vi "controller.vi"(11 "Shared_strings":string[][](array[string])) -> ()   [LabVIEW 2018]
uses:
  Global Variables.vi
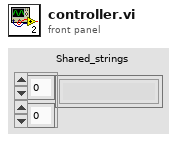
[diagram p1: front panel]
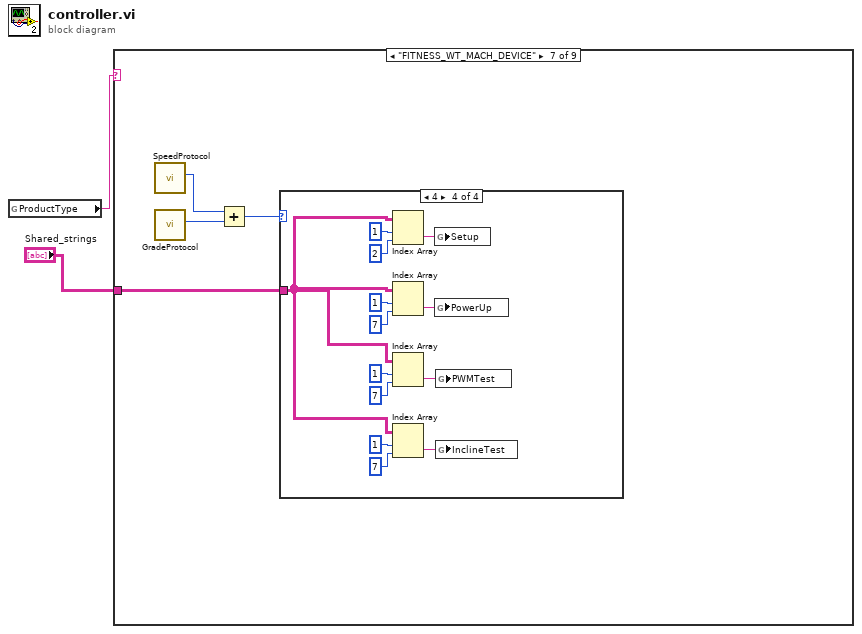
[diagram p0: block diagram]
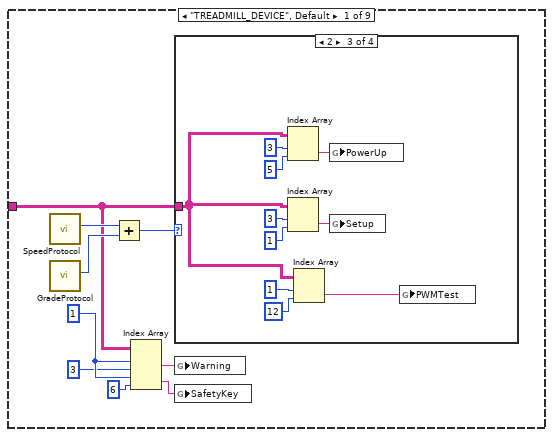
[diagram p2: hidden frame]
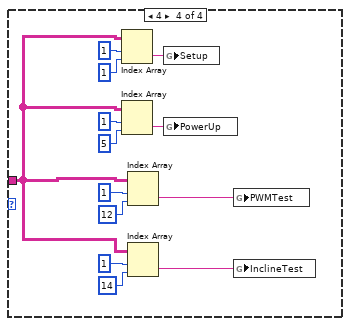
[diagram p5: hidden frame]
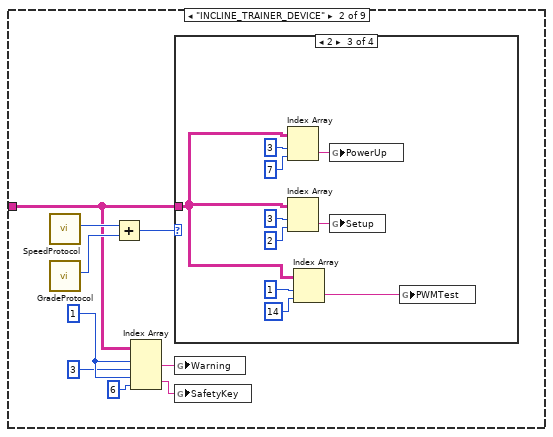
[diagram p6: hidden frame]
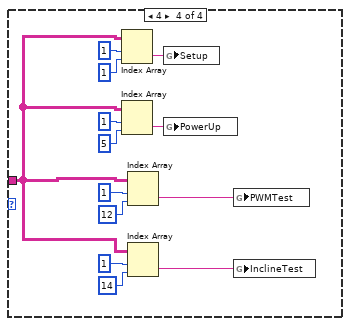
[diagram p9: hidden frame]
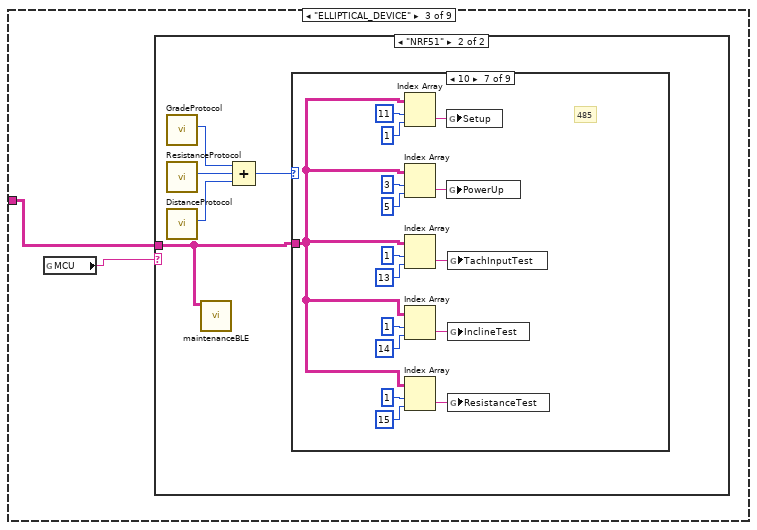
[diagram p10: hidden frame]
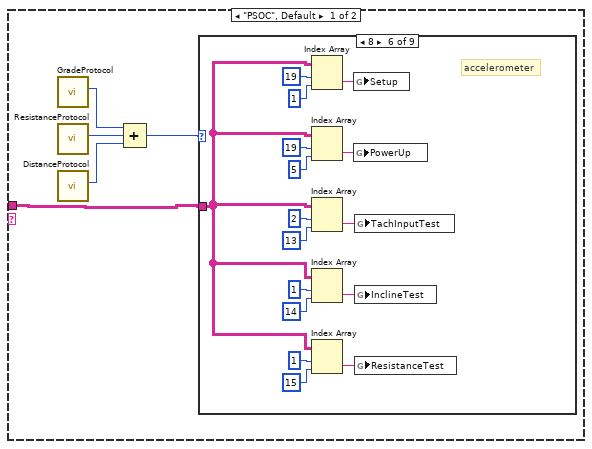
[diagram p11: hidden frame]
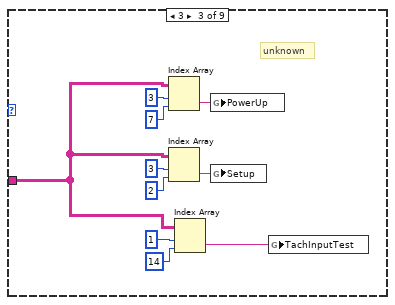
[diagram p14: hidden frame]
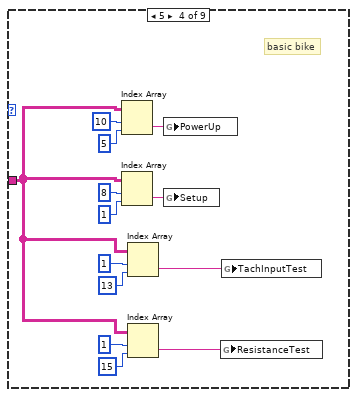
[diagram p15: hidden frame]
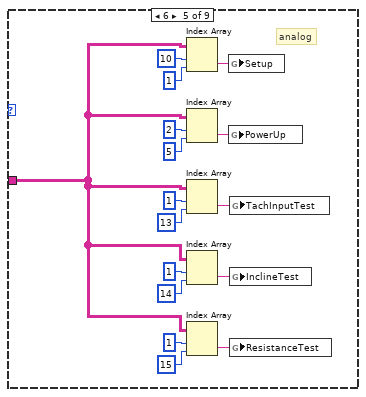
[diagram p16: hidden frame]
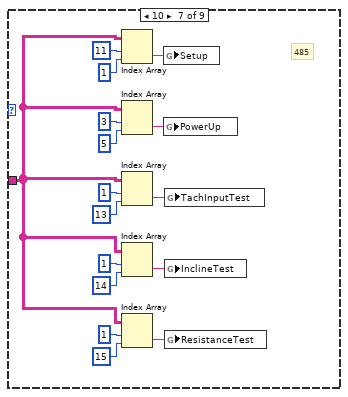
[diagram p17: hidden frame]
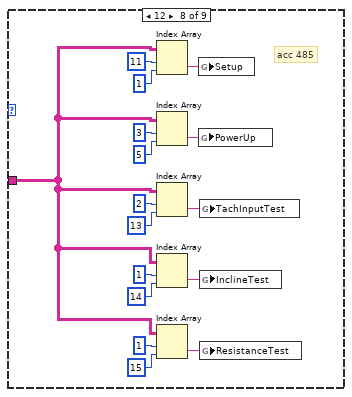
[diagram p18: hidden frame]
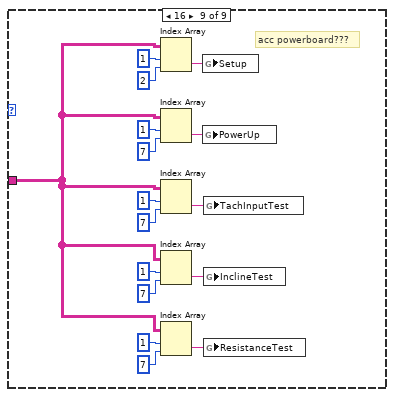
[diagram p19: hidden frame]
diagram:
  n1 = global read "Global Variables.vi" "ProductType"() -> (w1:string)
  n2 = case shown="\"FITNESS_WT_MACH_DEVICE\"" w1 {
    tunnel: "Shared_strings" -> [w3 w35 w68 w286 w406 w449 w667 w694 w913]
    frame "TREADMILL_DEVICE", Default {
      w8 = 1
      n3 = call "SpeedProtocol.vi"() -> ("output 1"=w11:i32)  [unwired: 9 in, 2 out]
      n4 = call "GradeProtocol.vi"() -> ("output 1"=w10:i32)  [unwired: 9 in, 2 out]
      n5 = Add(x=w11, y=w10) -> (x+y=w9:i32)
      n6 = Index Array(array=w3, index (row) #1=w8, index (col) #1=3, index (row) #2=w8, index (col) #2=6) -> (element #1=w5:string, element #2=w4:string)
      n7 = case shown="2" w9 {
        tunnel: w3 -> [_ _ w12 w22]
        frame 0, Default {
        }
        frame 1 {
        }
        frame 2 {
          n8 = Index Array(array=w12, index (row)=3, index (col)=5 ("disabled index (col)")) -> (element=w16:string)
          n9 = Index Array(array=w12, index (row)=3, index (col)=1 ("disabled index (col)")) -> (element=w21:string)
          n10 = Index Array(array=w12, index (row)=1, index (col)=12 ("disabled index (col)")) -> (element=w13:string)
          n11 = global write "Global Variables.vi" "PowerUp"(w16) -> ()
          n12 = global write "Global Variables.vi" "Setup"(w21) -> ()
          n13 = global write "Global Variables.vi" "PWMTest"(w13) -> ()
        }
        frame 4 {
          n14 = Index Array(array=w22, index (row)=1, index (col)=1 ("disabled index (col)")) -> (element=w34:string)
          n15 = Index Array(array=w22, index (row)=1, index (col)=5 ("disabled index (col)")) -> (element=w29:string)
          n16 = Index Array(array=w22, index (row)=1, index (col)=12 ("disabled index (col)")) -> (element=w26:string)
          n17 = Index Array(array=w22, index (row)=1, index (col)=14 ("disabled index (col)")) -> (element=w25:string)
          n18 = global write "Global Variables.vi" "Setup"(w34) -> ()
          n19 = global write "Global Variables.vi" "PowerUp"(w29) -> ()
          n20 = global write "Global Variables.vi" "PWMTest"(w26) -> ()
          n21 = global write "Global Variables.vi" "InclineTest"(w25) -> ()
        }
      }
      n22 = global write "Global Variables.vi" "Warning"(w5) -> ()
      n23 = global write "Global Variables.vi" "SafetyKey"(w4) -> ()
    }
    frame "INCLINE_TRAINER_DEVICE" {
      w40 = 1
      n24 = call "SpeedProtocol.vi"() -> ("output 1"=w43:i32)  [unwired: 9 in, 2 out]
      n25 = call "GradeProtocol.vi"() -> ("output 1"=w42:i32)  [unwired: 9 in, 2 out]
      n26 = Add(x=w43, y=w42) -> (x+y=w41:i32)
      n27 = Index Array(array=w35, index (row) #1=w40, index (col) #1=3, index (row) #2=w40, index (col) #2=6) -> (element #1=w36:string, element #2=w37:string)
      n28 = case shown="2" w41 {
        tunnel: w35 -> [_ _ w44 w54]
        frame 0, Default {
        }
        frame 1 {
        }
        frame 2 {
          n29 = Index Array(array=w44, index (row)=3, index (col)=7 ("disabled index (col)")) -> (element=w48:string)
          n30 = Index Array(array=w44, index (row)=3, index (col)=2 ("disabled index (col)")) -> (element=w53:string)
          n31 = Index Array(array=w44, index (row)=1, index (col)=14 ("disabled index (col)")) -> (element=w45:string)
          n32 = global write "Global Variables.vi" "PowerUp"(w48) -> ()
          n33 = global write "Global Variables.vi" "Setup"(w53) -> ()
          n34 = global write "Global Variables.vi" "PWMTest"(w45) -> ()
        }
        frame 4 {
          n35 = Index Array(array=w54, index (row)=1, index (col)=1 ("disabled index (col)")) -> (element=w66:string)
          n36 = Index Array(array=w54, index (row)=1, index (col)=5 ("disabled index (col)")) -> (element=w61:string)
          n37 = Index Array(array=w54, index (row)=1, index (col)=12 ("disabled index (col)")) -> (element=w58:string)
          n38 = Index Array(array=w54, index (row)=1, index (col)=14 ("disabled index (col)")) -> (element=w57:string)
          n39 = global write "Global Variables.vi" "Setup"(w66) -> ()
          n40 = global write "Global Variables.vi" "PowerUp"(w61) -> ()
          n41 = global write "Global Variables.vi" "PWMTest"(w58) -> ()
          n42 = global write "Global Variables.vi" "InclineTest"(w57) -> ()
        }
      }
      n43 = global write "Global Variables.vi" "Warning"(w36) -> ()
      n44 = global write "Global Variables.vi" "SafetyKey"(w37) -> ()
    }
    frame "ELLIPTICAL_DEVICE" {
      n45 = global read "Global Variables.vi" "MCU"() -> (w67:string)
      n46 = case shown="\"NRF51\"" w67 {
        tunnel: w68 -> [w70 w177]
        frame "PSOC", Default {
          n47 = call "GradeProtocol.vi"() -> ("output 1"=w71:i32)  [unwired: 9 in, 2 out]
          n48 = call "ResistanceProtocol.vi"() -> ("output 1"=w72:i32)  [unwired: 9 in, 2 out]
          n49 = call "DistanceProtocol.vi"() -> ("output 1"=w73:i32)  [unwired: 9 in, 2 out]
          n50 = Compound Arithmetic op=ADD(w71, w72, w73) -> (w69:i32)
          n51 = case shown="8" w69 {
            tunnel: w70 -> [_ _ w74 w84 w97 w113 w129 w145 w161]
            frame 0, Default {
            }
            frame 1 {
            }
            frame 3 {
              # "unknown"
              n52 = Index Array(array=w74, index (row)=3, index (col)=7 ("disabled index (col)")) -> (element=w78:string)
              n53 = Index Array(array=w74, index (row)=3, index (col)=2 ("disabled index (col)")) -> (element=w83:string)
              n54 = Index Array(array=w74, index (row)=1, index (col)=14 ("disabled index (col)")) -> (element=w75:string)
              n55 = global write "Global Variables.vi" "PowerUp"(w78) -> ()
              n56 = global write "Global Variables.vi" "Setup"(w83) -> ()
              n57 = global write "Global Variables.vi" "TachInputTest"(w75) -> ()
            }
            frame 5 {
              # "basic bike"
              n58 = Index Array(array=w84, index (row)=10, index (col)=5 ("disabled index (col)")) -> (element=w91:string)
              n59 = Index Array(array=w84, index (row)=8, index (col)=1 ("disabled index (col)")) -> (element=w96:string)
              n60 = Index Array(array=w84, index (row)=1, index (col)=13 ("disabled index (col)")) -> (element=w88:string)
              n61 = Index Array(array=w84, index (row)=1, index (col)=15 ("disabled index (col)")) -> (element=w87:string)
              n62 = global write "Global Variables.vi" "PowerUp"(w91) -> ()
              n63 = global write "Global Variables.vi" "Setup"(w96) -> ()
              n64 = global write "Global Variables.vi" "ResistanceTest"(w87) -> ()
              n65 = global write "Global Variables.vi" "TachInputTest"(w88) -> ()
            }
            frame 6 {
              # "analog"
              n66 = Index Array(array=w97, index (row)=10, index (col)=1 ("disabled index (col)")) -> (element=w112:string)
              n67 = Index Array(array=w97, index (row)=2, index (col)=5 ("disabled index (col)")) -> (element=w107:string)
              n68 = Index Array(array=w97, index (row)=1, index (col)=13 ("disabled index (col)")) -> (element=w104:string)
              n69 = Index Array(array=w97, index (row)=1, index (col)=14 ("disabled index (col)")) -> (element=w103:string)
              n70 = Index Array(array=w97, index (row)=1, index (col)=15 ("disabled index (col)")) -> (element=w98:string)
              n71 = global write "Global Variables.vi" "Setup"(w112) -> ()
              n72 = global write "Global Variables.vi" "PowerUp"(w107) -> ()
              n73 = global write "Global Variables.vi" "TachInputTest"(w104) -> ()
              n74 = global write "Global Variables.vi" "InclineTest"(w103) -> ()
              n75 = global write "Global Variables.vi" "ResistanceTest"(w98) -> ()
            }
            frame 8 {
              # "accelerometer"
              n76 = Index Array(array=w113, index (row)=19, index (col)=1 ("disabled index (col)")) -> (element=w128:string)
              n77 = Index Array(array=w113, index (row)=19, index (col)=5 ("disabled index (col)")) -> (element=w123:string)
              n78 = Index Array(array=w113, index (row)=2, index (col)=13 ("disabled index (col)")) -> (element=w120:string)
              n79 = Index Array(array=w113, index (row)=1, index (col)=14 ("disabled index (col)")) -> (element=w119:string)
              n80 = Index Array(array=w113, index (row)=1, index (col)=15 ("disabled index (col)")) -> (element=w114:string)
              n81 = global write "Global Variables.vi" "Setup"(w128) -> ()
              n82 = global write "Global Variables.vi" "PowerUp"(w123) -> ()
              n83 = global write "Global Variables.vi" "TachInputTest"(w120) -> ()
              n84 = global write "Global Variables.vi" "InclineTest"(w119) -> ()
              n85 = global write "Global Variables.vi" "ResistanceTest"(w114) -> ()
            }
            frame 10 {
              # "485"
              n86 = Index Array(array=w129, index (row)=11, index (col)=1 ("disabled index (col)")) -> (element=w144:string)
              n87 = Index Array(array=w129, index (row)=3, index (col)=5 ("disabled index (col)")) -> (element=w139:string)
              n88 = Index Array(array=w129, index (row)=1, index (col)=13 ("disabled index (col)")) -> (element=w136:string)
              n89 = Index Array(array=w129, index (row)=1, index (col)=14 ("disabled index (col)")) -> (element=w135:string)
              n90 = Index Array(array=w129, index (row)=1, index (col)=15 ("disabled index (col)")) -> (element=w130:string)
              n91 = global write "Global Variables.vi" "Setup"(w144) -> ()
              n92 = global write "Global Variables.vi" "PowerUp"(w139) -> ()
              n93 = global write "Global Variables.vi" "TachInputTest"(w136) -> ()
              n94 = global write "Global Variables.vi" "InclineTest"(w135) -> ()
              n95 = global write "Global Variables.vi" "ResistanceTest"(w130) -> ()
            }
            frame 12 {
              # "acc 485"
              n96 = Index Array(array=w145, index (row)=11, index (col)=1 ("disabled index (col)")) -> (element=w160:string)
              n97 = Index Array(array=w145, index (row)=3, index (col)=5 ("disabled index (col)")) -> (element=w155:string)
              n98 = Index Array(array=w145, index (row)=2, index (col)=13 ("disabled index (col)")) -> (element=w152:string)
              n99 = Index Array(array=w145, index (row)=1, index (col)=14 ("disabled index (col)")) -> (element=w151:string)
              n100 = Index Array(array=w145, index (row)=1, index (col)=15 ("disabled index (col)")) -> (element=w146:string)
              n101 = global write "Global Variables.vi" "Setup"(w160) -> ()
              n102 = global write "Global Variables.vi" "PowerUp"(w155) -> ()
              n103 = global write "Global Variables.vi" "TachInputTest"(w152) -> ()
              n104 = global write "Global Variables.vi" "InclineTest"(w151) -> ()
              n105 = global write "Global Variables.vi" "ResistanceTest"(w146) -> ()
            }
            frame 16 {
              # "acc powerboard???"
              n106 = Index Array(array=w161, index (row)=1, index (col)=2 ("disabled index (col)")) -> (element=w176:string)
              n107 = Index Array(array=w161, index (row)=1, index (col)=7 ("disabled index (col)")) -> (element=w171:string)
              n108 = Index Array(array=w161, index (row)=1, index (col)=7 ("disabled index (col)")) -> (element=w168:string)
              n109 = Index Array(array=w161, index (row)=1, index (col)=7 ("disabled index (col)")) -> (element=w167:string)
              n110 = Index Array(array=w161, index (row)=1, index (col)=7 ("disabled index (col)")) -> (element=w162:string)
              n111 = global write "Global Variables.vi" "Setup"(w176) -> ()
              n112 = global write "Global Variables.vi" "PowerUp"(w171) -> ()
              n113 = global write "Global Variables.vi" "TachInputTest"(w168) -> ()
              n114 = global write "Global Variables.vi" "InclineTest"(w167) -> ()
              n115 = global write "Global Variables.vi" "ResistanceTest"(w162) -> ()
            }
          }
        }
        frame "NRF51" {
          n116 = call "GradeProtocol.vi"() -> ("output 1"=w179:i32)  [unwired: 9 in, 2 out]
          n117 = call "ResistanceProtocol.vi"() -> ("output 1"=w180:i32)  [unwired: 9 in, 2 out]
          n118 = call "DistanceProtocol.vi"() -> ("output 1"=w181:i32)  [unwired: 9 in, 2 out]
          n119 = call "maintenanceBLE.vi"("Shared_strings"=w177) -> ()  [unwired: 11 in]
          n120 = Compound Arithmetic op=ADD(w179, w180, w181) -> (w178:i32)
          n121 = case shown="10" w178 {
            tunnel: w177 -> [_ _ w182 w192 w205 w221 w237 w253 w269]
            frame 0, Default {
            }
            frame 1 {
            }
            frame 3 {
              # "unknown"
              n122 = Index Array(array=w182, index (row)=3, index (col)=7 ("disabled index (col)")) -> (element=w186:string)
              n123 = Index Array(array=w182, index (row)=3, index (col)=2 ("disabled index (col)")) -> (element=w191:string)
              n124 = Index Array(array=w182, index (row)=1, index (col)=14 ("disabled index (col)")) -> (element=w183:string)
              n125 = global write "Global Variables.vi" "PowerUp"(w186) -> ()
              n126 = global write "Global Variables.vi" "Setup"(w191) -> ()
              n127 = global write "Global Variables.vi" "TachInputTest"(w183) -> ()
            }
            frame 5 {
              # "basic bike"
              n128 = Index Array(array=w192, index (row)=10, index (col)=5 ("disabled index (col)")) -> (element=w199:string)
              n129 = Index Array(array=w192, index (row)=8, index (col)=1 ("disabled index (col)")) -> (element=w204:string)
              n130 = Index Array(array=w192, index (row)=1, index (col)=13 ("disabled index (col)")) -> (element=w196:string)
              n131 = Index Array(array=w192, index (row)=1, index (col)=15 ("disabled index (col)")) -> (element=w195:string)
              n132 = global write "Global Variables.vi" "PowerUp"(w199) -> ()
              n133 = global write "Global Variables.vi" "Setup"(w204) -> ()
              n134 = global write "Global Variables.vi" "ResistanceTest"(w195) -> ()
              n135 = global write "Global Variables.vi" "TachInputTest"(w196) -> ()
            }
            frame 6 {
              # "analog"
              n136 = Index Array(array=w205, index (row)=10, index (col)=1 ("disabled index (col)")) -> (element=w220:string)
              n137 = Index Array(array=w205, index (row)=2, index (col)=5 ("disabled index (col)")) -> (element=w215:string)
              n138 = Index Array(array=w205, index (row)=1, index (col)=13 ("disabled index (col)")) -> (element=w212:string)
              n139 = Index Array(array=w205, index (row)=1, index (col)=14 ("disabled index (col)")) -> (element=w211:string)
              n140 = Index Array(array=w205, index (row)=1, index (col)=15 ("disabled index (col)")) -> (element=w206:string)
              n141 = global write "Global Variables.vi" "Setup"(w220) -> ()
              n142 = global write "Global Variables.vi" "PowerUp"(w215) -> ()
              n143 = global write "Global Variables.vi" "TachInputTest"(w212) -> ()
              n144 = global write "Global Variables.vi" "InclineTest"(w211) -> ()
              n145 = global write "Global Variables.vi" "ResistanceTest"(w206) -> ()
            }
            frame 8 {
              # "accelerometer"
              n146 = Index Array(array=w221, index (row)=19, index (col)=1 ("disabled index (col)")) -> (element=w236:string)
              n147 = Index Array(array=w221, index (row)=19, index (col)=5 ("disabled index (col)")) -> (element=w231:string)
              n148 = Index Array(array=w221, index (row)=2, index (col)=13 ("disabled index (col)")) -> (element=w228:string)
              n149 = Index Array(array=w221, index (row)=1, index (col)=14 ("disabled index (col)")) -> (element=w227:string)
              n150 = Index Array(array=w221, index (row)=1, index (col)=15 ("disabled index (col)")) -> (element=w222:string)
              n151 = global write "Global Variables.vi" "Setup"(w236) -> ()
              n152 = global write "Global Variables.vi" "PowerUp"(w231) -> ()
              n153 = global write "Global Variables.vi" "TachInputTest"(w228) -> ()
              n154 = global write "Global Variables.vi" "InclineTest"(w227) -> ()
              n155 = global write "Global Variables.vi" "ResistanceTest"(w222) -> ()
            }
            frame 10 {
              # "485"
              n156 = Index Array(array=w237, index (row)=11, index (col)=1 ("disabled index (col)")) -> (element=w252:string)
              n157 = Index Array(array=w237, index (row)=3, index (col)=5 ("disabled index (col)")) -> (element=w247:string)
              n158 = Index Array(array=w237, index (row)=1, index (col)=13 ("disabled index (col)")) -> (element=w244:string)
              n159 = Index Array(array=w237, index (row)=1, index (col)=14 ("disabled index (col)")) -> (element=w243:string)
              n160 = Index Array(array=w237, index (row)=1, index (col)=15 ("disabled index (col)")) -> (element=w238:string)
              n161 = global write "Global Variables.vi" "Setup"(w252) -> ()
              n162 = global write "Global Variables.vi" "PowerUp"(w247) -> ()
              n163 = global write "Global Variables.vi" "TachInputTest"(w244) -> ()
              n164 = global write "Global Variables.vi" "InclineTest"(w243) -> ()
              n165 = global write "Global Variables.vi" "ResistanceTest"(w238) -> ()
            }
            frame 12 {
              # "acc 485"
              n166 = Index Array(array=w253, index (row)=11, index (col)=1 ("disabled index (col)")) -> (element=w268:string)
              n167 = Index Array(array=w253, index (row)=3, index (col)=5 ("disabled index (col)")) -> (element=w263:string)
              n168 = Index Array(array=w253, index (row)=2, index (col)=13 ("disabled index (col)")) -> (element=w260:string)
              n169 = Index Array(array=w253, index (row)=1, index (col)=14 ("disabled index (col)")) -> (element=w259:string)
              n170 = Index Array(array=w253, index (row)=1, index (col)=15 ("disabled index (col)")) -> (element=w254:string)
              n171 = global write "Global Variables.vi" "Setup"(w268) -> ()
              n172 = global write "Global Variables.vi" "PowerUp"(w263) -> ()
              n173 = global write "Global Variables.vi" "TachInputTest"(w260) -> ()
              n174 = global write "Global Variables.vi" "InclineTest"(w259) -> ()
              n175 = global write "Global Variables.vi" "ResistanceTest"(w254) -> ()
            }
            frame 16 {
              # "acc powerboard???"
              n176 = Index Array(array=w269, index (row)=1, index (col)=2 ("disabled index (col)")) -> (element=w284:string)
              n177 = Index Array(array=w269, index (row)=1, index (col)=7 ("disabled index (col)")) -> (element=w279:string)
              n178 = Index Array(array=w269, index (row)=1, index (col)=7 ("disabled index (col)")) -> (element=w276:string)
              n179 = Index Array(array=w269, index (row)=1, index (col)=7 ("disabled index (col)")) -> (element=w275:string)
              n180 = Index Array(array=w269, index (row)=1, index (col)=7 ("disabled index (col)")) -> (element=w270:string)
              n181 = global write "Global Variables.vi" "Setup"(w284) -> ()
              n182 = global write "Global Variables.vi" "PowerUp"(w279) -> ()
              n183 = global write "Global Variables.vi" "TachInputTest"(w276) -> ()
              n184 = global write "Global Variables.vi" "InclineTest"(w275) -> ()
              n185 = global write "Global Variables.vi" "ResistanceTest"(w270) -> ()
            }
          }
        }
      }
    }
    frame "EXERCISE_BIKE_DEVICE" {
      n186 = global read "Global Variables.vi" "MCU"() -> (w285:string)
      n187 = case shown="\"PSOC\", Default" w285 {
        tunnel: w286 -> [w287 w346]
        frame "PSOC", Default {
          n188 = call "GradeProtocol.vi"() -> ("output 1"=w290:i32)  [unwired: 9 in, 2 out]
          n189 = call "ResistanceProtocol.vi"() -> ("output 1"=w289:i32)  [unwired: 9 in, 2 out]
          n190 = Compound Arithmetic op=ADD(w290, w289) -> (w288:i32)
          n191 = case shown="3" w288 {
            tunnel: w287 -> [_ _ w291 w301 w314 w330]
            frame 0, Default {
            }
            frame 1 {
            }
            frame 2 {
              # "incomplete"
              n192 = Index Array(array=w291, index (row)=3, index (col)=5 ("disabled index (col)")) -> (element=w295:string)
              n193 = Index Array(array=w291, index (row)=14, index (col)=1 ("disabled index (col)")) -> (element=w300:string)
              n194 = Index Array(array=w291, index (row)=1, index (col)=14 ("disabled index (col)")) -> (element=w292:string)
              n195 = global write "Global Variables.vi" "PowerUp"(w295) -> ()
              n196 = global write "Global Variables.vi" "Setup"(w300) -> ()
              n197 = global write "Global Variables.vi" "TachInputTest"(w292) -> ()
            }
            frame 3 {
              # "basic bike"
              n198 = Index Array(array=w301, index (row)=8, index (col)=1 ("disabled index (col)")) -> (element=w313:string)
              n199 = Index Array(array=w301, index (row)=8, index (col)=5 ("disabled index (col)")) -> (element=w308:string)
              n200 = Index Array(array=w301, index (row)=1, index (col)=13 ("disabled index (col)")) -> (element=w305:string)
              n201 = Index Array(array=w301, index (row)=1, index (col)=15 ("disabled index (col)")) -> (element=w304:string)
              n202 = global write "Global Variables.vi" "TachInputTest"(w305) -> ()
              n203 = global write "Global Variables.vi" "ResistanceTest"(w304) -> ()
              n204 = global write "Global Variables.vi" "Setup"(w313) -> ()
              n205 = global write "Global Variables.vi" "PowerUp"(w308) -> ()
            }
            frame 4 {
              # "analog"
              n206 = Index Array(array=w314, index (row)=9, index (col)=1 ("disabled index (col)")) -> (element=w329:string)
              n207 = Index Array(array=w314, index (row)=8, index (col)=5 ("disabled index (col)")) -> (element=w324:string)
              n208 = Index Array(array=w314, index (row)=1, index (col)=13 ("disabled index (col)")) -> (element=w321:string)
              n209 = Index Array(array=w314, index (row)=1, index (col)=14 ("disabled index (col)")) -> (element=w320:string)
              n210 = Index Array(array=w314, index (row)=1, index (col)=15 ("disabled index (col)")) -> (element=w315:string)
              n211 = global write "Global Variables.vi" "TachInputTest"(w321) -> ()
              n212 = global write "Global Variables.vi" "ResistanceTest"(w315) -> ()
              n213 = global write "Global Variables.vi" "Setup"(w329) -> ()
              n214 = global write "Global Variables.vi" "PowerUp"(w324) -> ()
              n215 = global write "Global Variables.vi" "InclineTest"(w320) -> ()
            }
            frame 8 {
              # "485"
              n216 = Index Array(array=w330, index (row)=11, index (col)=1 ("disabled index (col)")) -> (element=w345:string)
              n217 = Index Array(array=w330, index (row)=3, index (col)=5 ("disabled index (col)")) -> (element=w340:string)
              n218 = Index Array(array=w330, index (row)=1, index (col)=13 ("disabled index (col)")) -> (element=w337:string)
              n219 = Index Array(array=w330, index (row)=1, index (col)=14 ("disabled index (col)")) -> (element=w336:string)
              n220 = Index Array(array=w330, index (row)=1, index (col)=15 ("disabled index (col)")) -> (element=w331:string)
              n221 = global write "Global Variables.vi" "TachInputTest"(w337) -> ()
              n222 = global write "Global Variables.vi" "ResistanceTest"(w331) -> ()
              n223 = global write "Global Variables.vi" "Setup"(w345) -> ()
              n224 = global write "Global Variables.vi" "PowerUp"(w340) -> ()
              n225 = global write "Global Variables.vi" "InclineTest"(w336) -> ()
            }
          }
        }
        frame "NRF51" {
          n226 = call "GradeProtocol.vi"() -> ("output 1"=w349:i32)  [unwired: 9 in, 2 out]
          n227 = call "ResistanceProtocol.vi"() -> ("output 1"=w348:i32)  [unwired: 9 in, 2 out]
          n228 = call "maintenanceBLE.vi"("Shared_strings"=w346) -> ()  [unwired: 11 in]
          n229 = Compound Arithmetic op=ADD(w349, w348) -> (w347:i32)
          n230 = case shown="3" w347 {
            tunnel: w346 -> [_ _ w350 w360 w373 w389]
            frame 0, Default {
            }
            frame 1 {
            }
            frame 2 {
              # "incomplete"
              n231 = Index Array(array=w350, index (row)=3, index (col)=5 ("disabled index (col)")) -> (element=w354:string)
              n232 = Index Array(array=w350, index (row)=14, index (col)=1 ("disabled index (col)")) -> (element=w359:string)
              n233 = Index Array(array=w350, index (row)=1, index (col)=14 ("disabled index (col)")) -> (element=w351:string)
              n234 = global write "Global Variables.vi" "PowerUp"(w354) -> ()
              n235 = global write "Global Variables.vi" "Setup"(w359) -> ()
              n236 = global write "Global Variables.vi" "TachInputTest"(w351) -> ()
            }
            frame 3 {
              n237 = Index Array(array=w360, index (row)=8, index (col)=1 ("disabled index (col)")) -> (element=w372:string)
              n238 = Index Array(array=w360, index (row)=8, index (col)=5 ("disabled index (col)")) -> (element=w367:string)
              n239 = Index Array(array=w360, index (row)=1, index (col)=13 ("disabled index (col)")) -> (element=w364:string)
              n240 = Index Array(array=w360, index (row)=1, index (col)=15 ("disabled index (col)")) -> (element=w363:string)
              n241 = global write "Global Variables.vi" "TachInputTest"(w364) -> ()
              n242 = global write "Global Variables.vi" "ResistanceTest"(w363) -> ()
              n243 = global write "Global Variables.vi" "Setup"(w372) -> ()
              n244 = global write "Global Variables.vi" "PowerUp"(w367) -> ()
            }
            frame 4 {
              # "analog"
              n245 = Index Array(array=w373, index (row)=9, index (col)=1 ("disabled index (col)")) -> (element=w388:string)
              n246 = Index Array(array=w373, index (row)=8, index (col)=5 ("disabled index (col)")) -> (element=w383:string)
              n247 = Index Array(array=w373, index (row)=1, index (col)=13 ("disabled index (col)")) -> (element=w380:string)
              n248 = Index Array(array=w373, index (row)=1, index (col)=14 ("disabled index (col)")) -> (element=w379:string)
              n249 = Index Array(array=w373, index (row)=1, index (col)=15 ("disabled index (col)")) -> (element=w374:string)
              n250 = global write "Global Variables.vi" "TachInputTest"(w380) -> ()
              n251 = global write "Global Variables.vi" "ResistanceTest"(w374) -> ()
              n252 = global write "Global Variables.vi" "Setup"(w388) -> ()
              n253 = global write "Global Variables.vi" "PowerUp"(w383) -> ()
              n254 = global write "Global Variables.vi" "InclineTest"(w379) -> ()
            }
            frame 8 {
              # "485"
              n255 = Index Array(array=w389, index (row)=11, index (col)=1 ("disabled index (col)")) -> (element=w404:string)
              n256 = Index Array(array=w389, index (row)=3, index (col)=5 ("disabled index (col)")) -> (element=w399:string)
              n257 = Index Array(array=w389, index (row)=1, index (col)=13 ("disabled index (col)")) -> (element=w396:string)
              n258 = Index Array(array=w389, index (row)=1, index (col)=14 ("disabled index (col)")) -> (element=w395:string)
              n259 = Index Array(array=w389, index (row)=1, index (col)=15 ("disabled index (col)")) -> (element=w390:string)
              n260 = global write "Global Variables.vi" "TachInputTest"(w396) -> ()
              n261 = global write "Global Variables.vi" "ResistanceTest"(w390) -> ()
              n262 = global write "Global Variables.vi" "Setup"(w404) -> ()
              n263 = global write "Global Variables.vi" "PowerUp"(w399) -> ()
              n264 = global write "Global Variables.vi" "InclineTest"(w395) -> ()
            }
          }
        }
      }
    }
    frame "SPIN_BIKE_DEVICE" {
      n265 = global read "Global Variables.vi" "MCU"() -> (w405:string)
      n266 = case shown="\"NRF51\", Default" w405 {
        tunnel: w406 -> [w407 w429]
        frame "NRF51", Default {
          n267 = call "maintenanceBLE.vi"("Shared_strings"=w407) -> ()  [unwired: 11 in]
          n268 = call "SpeedProtocol.vi"() -> ("output 1"=w411:i32)  [unwired: 9 in, 2 out]
          n269 = call "GradeProtocol.vi"() -> ("output 1"=w410:i32)  [unwired: 9 in, 2 out]
          n270 = call "ResistanceProtocol.vi"() -> ("output 1"=w408:i32)  [unwired: 9 in, 2 out]
          n271 = Compound Arithmetic op=ADD(w411, w410, w408) -> (w409:i32)
          n272 = case shown="12" w409 {
            tunnel: w407 -> [_ w412]
            frame 0, Default {
            }
            frame 12 {
              # "RS485"
              n273 = Index Array(array=w412, index (row)=3, index (col)=5 ("disabled index (col)")) -> (element=w422:string)
              n274 = Index Array(array=w412, index (row)=1, index (col)=13 ("disabled index (col)")) -> (element=w419:string)
              n275 = Index Array(array=w412, index (row)=11, index (col)=1 ("disabled index (col)")) -> (element=w427:string)
              n276 = Index Array(array=w412, index (row)=1, index (col)=14 ("disabled index (col)")) -> (element=w418:string)
              n277 = Index Array(array=w412, index (row)=1, index (col)=15 ("disabled index (col)")) -> (element=w413:string)
              n278 = global write "Global Variables.vi" "PowerUp"(w422) -> ()
              n279 = global write "Global Variables.vi" "Setup"(w427) -> ()
              n280 = global write "Global Variables.vi" "TachInputTest"(w419) -> ()
              n281 = global write "Global Variables.vi" "InclineTest"(w418) -> ()
              n282 = global write "Global Variables.vi" "ResistanceTest"(w413) -> ()
            }
          }
        }
        frame "PSOC" {
          n283 = call "SpeedProtocol.vi"() -> ("output 1"=w432:i32)  [unwired: 9 in, 2 out]
          n284 = call "GradeProtocol.vi"() -> ("output 1"=w431:i32)  [unwired: 9 in, 2 out]
          n285 = call "ResistanceProtocol.vi"() -> ("output 1"=w428:i32)  [unwired: 9 in, 2 out]
          n286 = Compound Arithmetic op=ADD(w432, w431, w428) -> (w430:i32)
          n287 = case shown="12" w430 {
            tunnel: w429 -> [_ w433]
            frame 0, Default {
            }
            frame 12 {
              # "RS485"
              n288 = Index Array(array=w433, index (row)=16, index (col)=1 ("disabled index (col)")) -> (element=w448:string)
              n289 = Index Array(array=w433, index (row)=16, index (col)=5 ("disabled index (col)")) -> (element=w443:string)
              n290 = Index Array(array=w433, index (row)=1, index (col)=13 ("disabled index (col)")) -> (element=w440:string)
              n291 = Index Array(array=w433, index (row)=1, index (col)=14 ("disabled index (col)")) -> (element=w439:string)
              n292 = Index Array(array=w433, index (row)=1, index (col)=15 ("disabled index (col)")) -> (element=w434:string)
              n293 = global write "Global Variables.vi" "Setup"(w448) -> ()
              n294 = global write "Global Variables.vi" "PowerUp"(w443) -> ()
              n295 = global write "Global Variables.vi" "TachInputTest"(w440) -> ()
              n296 = global write "Global Variables.vi" "InclineTest"(w439) -> ()
              n297 = global write "Global Variables.vi" "ResistanceTest"(w434) -> ()
            }
          }
        }
      }
    }
    frame "VERTICAL_ELLIPTICAL_DEVICE" {
      n298 = global read "Global Variables.vi" "MCU"() -> (w450:string)
      n299 = case shown="\"NRF51\"" w450 {
        tunnel: w449 -> [w452 w559]
        frame "PSOC", Default {
          n300 = call "GradeProtocol.vi"() -> ("output 1"=w453:i32)  [unwired: 9 in, 2 out]
          n301 = call "ResistanceProtocol.vi"() -> ("output 1"=w454:i32)  [unwired: 9 in, 2 out]
          n302 = call "DistanceProtocol.vi"() -> ("output 1"=w455:i32)  [unwired: 9 in, 2 out]
          n303 = Compound Arithmetic op=ADD(w453, w454, w455) -> (w451:i32)
          n304 = case shown="8" w451 {
            tunnel: w452 -> [_ _ w456 w466 w479 w495 w511 w527 w543]
            frame 0, Default {
            }
            frame 1 {
            }
            frame 3 {
              # "unknown"
              n305 = Index Array(array=w456, index (row)=3, index (col)=7 ("disabled index (col)")) -> (element=w460:string)
              n306 = Index Array(array=w456, index (row)=3, index (col)=2 ("disabled index (col)")) -> (element=w465:string)
              n307 = Index Array(array=w456, index (row)=1, index (col)=14 ("disabled index (col)")) -> (element=w457:string)
              n308 = global write "Global Variables.vi" "PowerUp"(w460) -> ()
              n309 = global write "Global Variables.vi" "Setup"(w465) -> ()
              n310 = global write "Global Variables.vi" "TachInputTest"(w457) -> ()
            }
            frame 5 {
              # "basic bike"
              n311 = Index Array(array=w466, index (row)=10, index (col)=5 ("disabled index (col)")) -> (element=w473:string)
              n312 = Index Array(array=w466, index (row)=8, index (col)=1 ("disabled index (col)")) -> (element=w478:string)
              n313 = Index Array(array=w466, index (row)=1, index (col)=13 ("disabled index (col)")) -> (element=w470:string)
              n314 = Index Array(array=w466, index (row)=1, index (col)=15 ("disabled index (col)")) -> (element=w469:string)
              n315 = global write "Global Variables.vi" "PowerUp"(w473) -> ()
              n316 = global write "Global Variables.vi" "Setup"(w478) -> ()
              n317 = global write "Global Variables.vi" "ResistanceTest"(w469) -> ()
              n318 = global write "Global Variables.vi" "TachInputTest"(w470) -> ()
            }
            frame 6 {
              # "analog"
              n319 = Index Array(array=w479, index (row)=10, index (col)=1 ("disabled index (col)")) -> (element=w494:string)
              n320 = Index Array(array=w479, index (row)=2, index (col)=5 ("disabled index (col)")) -> (element=w489:string)
              n321 = Index Array(array=w479, index (row)=1, index (col)=13 ("disabled index (col)")) -> (element=w486:string)
              n322 = Index Array(array=w479, index (row)=1, index (col)=14 ("disabled index (col)")) -> (element=w485:string)
              n323 = Index Array(array=w479, index (row)=1, index (col)=15 ("disabled index (col)")) -> (element=w480:string)
              n324 = global write "Global Variables.vi" "Setup"(w494) -> ()
              n325 = global write "Global Variables.vi" "PowerUp"(w489) -> ()
              n326 = global write "Global Variables.vi" "TachInputTest"(w486) -> ()
              n327 = global write "Global Variables.vi" "InclineTest"(w485) -> ()
              n328 = global write "Global Variables.vi" "ResistanceTest"(w480) -> ()
            }
            frame 8 {
              # "accelerometer"
              n329 = Index Array(array=w495, index (row)=19, index (col)=1 ("disabled index (col)")) -> (element=w510:string)
              n330 = Index Array(array=w495, index (row)=19, index (col)=5 ("disabled index (col)")) -> (element=w505:string)
              n331 = Index Array(array=w495, index (row)=2, index (col)=13 ("disabled index (col)")) -> (element=w502:string)
              n332 = Index Array(array=w495, index (row)=1, index (col)=14 ("disabled index (col)")) -> (element=w501:string)
              n333 = Index Array(array=w495, index (row)=1, index (col)=15 ("disabled index (col)")) -> (element=w496:string)
              n334 = global write "Global Variables.vi" "Setup"(w510) -> ()
              n335 = global write "Global Variables.vi" "PowerUp"(w505) -> ()
              n336 = global write "Global Variables.vi" "TachInputTest"(w502) -> ()
              n337 = global write "Global Variables.vi" "InclineTest"(w501) -> ()
              n338 = global write "Global Variables.vi" "ResistanceTest"(w496) -> ()
            }
            frame 10 {
              # "485"
              n339 = Index Array(array=w511, index (row)=11, index (col)=1 ("disabled index (col)")) -> (element=w526:string)
              n340 = Index Array(array=w511, index (row)=3, index (col)=5 ("disabled index (col)")) -> (element=w521:string)
              n341 = Index Array(array=w511, index (row)=1, index (col)=13 ("disabled index (col)")) -> (element=w518:string)
              n342 = Index Array(array=w511, index (row)=1, index (col)=14 ("disabled index (col)")) -> (element=w517:string)
              n343 = Index Array(array=w511, index (row)=1, index (col)=15 ("disabled index (col)")) -> (element=w512:string)
              n344 = global write "Global Variables.vi" "Setup"(w526) -> ()
              n345 = global write "Global Variables.vi" "PowerUp"(w521) -> ()
              n346 = global write "Global Variables.vi" "TachInputTest"(w518) -> ()
              n347 = global write "Global Variables.vi" "InclineTest"(w517) -> ()
              n348 = global write "Global Variables.vi" "ResistanceTest"(w512) -> ()
            }
            frame 12 {
              # "acc 485"
              n349 = Index Array(array=w527, index (row)=11, index (col)=1 ("disabled index (col)")) -> (element=w542:string)
              n350 = Index Array(array=w527, index (row)=3, index (col)=5 ("disabled index (col)")) -> (element=w537:string)
              n351 = Index Array(array=w527, index (row)=2, index (col)=13 ("disabled index (col)")) -> (element=w534:string)
              n352 = Index Array(array=w527, index (row)=1, index (col)=14 ("disabled index (col)")) -> (element=w533:string)
              n353 = Index Array(array=w527, index (row)=1, index (col)=15 ("disabled index (col)")) -> (element=w528:string)
              n354 = global write "Global Variables.vi" "Setup"(w542) -> ()
              n355 = global write "Global Variables.vi" "PowerUp"(w537) -> ()
              n356 = global write "Global Variables.vi" "TachInputTest"(w534) -> ()
              n357 = global write "Global Variables.vi" "InclineTest"(w533) -> ()
              n358 = global write "Global Variables.vi" "ResistanceTest"(w528) -> ()
            }
            frame 16 {
              # "acc powerboard???"
              n359 = Index Array(array=w543, index (row)=1, index (col)=2 ("disabled index (col)")) -> (element=w558:string)
              n360 = Index Array(array=w543, index (row)=1, index (col)=7 ("disabled index (col)")) -> (element=w553:string)
              n361 = Index Array(array=w543, index (row)=1, index (col)=7 ("disabled index (col)")) -> (element=w550:string)
              n362 = Index Array(array=w543, index (row)=1, index (col)=7 ("disabled index (col)")) -> (element=w549:string)
              n363 = Index Array(array=w543, index (row)=1, index (col)=7 ("disabled index (col)")) -> (element=w544:string)
              n364 = global write "Global Variables.vi" "Setup"(w558) -> ()
              n365 = global write "Global Variables.vi" "PowerUp"(w553) -> ()
              n366 = global write "Global Variables.vi" "TachInputTest"(w550) -> ()
              n367 = global write "Global Variables.vi" "InclineTest"(w549) -> ()
              n368 = global write "Global Variables.vi" "ResistanceTest"(w544) -> ()
            }
          }
        }
        frame "NRF51" {
          n369 = call "GradeProtocol.vi"() -> ("output 1"=w561:i32)  [unwired: 9 in, 2 out]
          n370 = call "ResistanceProtocol.vi"() -> ("output 1"=w562:i32)  [unwired: 9 in, 2 out]
          n371 = call "DistanceProtocol.vi"() -> ("output 1"=w563:i32)  [unwired: 9 in, 2 out]
          n372 = call "maintenanceBLE.vi"("Shared_strings"=w559) -> ()  [unwired: 11 in]
          n373 = Compound Arithmetic op=ADD(w561, w562, w563) -> (w560:i32)
          n374 = case shown="10" w560 {
            tunnel: w559 -> [_ _ w564 w574 w587 w603 w619 w635 w651]
            frame 0, Default {
            }
            frame 1 {
            }
            frame 3 {
              # "unknown"
              n375 = Index Array(array=w564, index (row)=3, index (col)=7 ("disabled index (col)")) -> (element=w568:string)
              n376 = Index Array(array=w564, index (row)=3, index (col)=2 ("disabled index (col)")) -> (element=w573:string)
              n377 = Index Array(array=w564, index (row)=1, index (col)=14 ("disabled index (col)")) -> (element=w565:string)
              n378 = global write "Global Variables.vi" "PowerUp"(w568) -> ()
              n379 = global write "Global Variables.vi" "Setup"(w573) -> ()
              n380 = global write "Global Variables.vi" "TachInputTest"(w565) -> ()
            }
            frame 5 {
              # "basic bike"
              n381 = Index Array(array=w574, index (row)=10, index (col)=5 ("disabled index (col)")) -> (element=w581:string)
              n382 = Index Array(array=w574, index (row)=8, index (col)=1 ("disabled index (col)")) -> (element=w586:string)
              n383 = Index Array(array=w574, index (row)=1, index (col)=13 ("disabled index (col)")) -> (element=w578:string)
              n384 = Index Array(array=w574, index (row)=1, index (col)=15 ("disabled index (col)")) -> (element=w577:string)
              n385 = global write "Global Variables.vi" "PowerUp"(w581) -> ()
              n386 = global write "Global Variables.vi" "Setup"(w586) -> ()
              n387 = global write "Global Variables.vi" "ResistanceTest"(w577) -> ()
              n388 = global write "Global Variables.vi" "TachInputTest"(w578) -> ()
            }
            frame 6 {
              # "analog"
              n389 = Index Array(array=w587, index (row)=10, index (col)=1 ("disabled index (col)")) -> (element=w602:string)
              n390 = Index Array(array=w587, index (row)=2, index (col)=5 ("disabled index (col)")) -> (element=w597:string)
              n391 = Index Array(array=w587, index (row)=1, index (col)=13 ("disabled index (col)")) -> (element=w594:string)
              n392 = Index Array(array=w587, index (row)=1, index (col)=14 ("disabled index (col)")) -> (element=w593:string)
              n393 = Index Array(array=w587, index (row)=1, index (col)=15 ("disabled index (col)")) -> (element=w588:string)
              n394 = global write "Global Variables.vi" "Setup"(w602) -> ()
              n395 = global write "Global Variables.vi" "PowerUp"(w597) -> ()
              n396 = global write "Global Variables.vi" "TachInputTest"(w594) -> ()
              n397 = global write "Global Variables.vi" "InclineTest"(w593) -> ()
              n398 = global write "Global Variables.vi" "ResistanceTest"(w588) -> ()
            }
            frame 8 {
              # "accelerometer"
              n399 = Index Array(array=w603, index (row)=19, index (col)=1 ("disabled index (col)")) -> (element=w618:string)
              n400 = Index Array(array=w603, index (row)=19, index (col)=5 ("disabled index (col)")) -> (element=w613:string)
              n401 = Index Array(array=w603, index (row)=2, index (col)=13 ("disabled index (col)")) -> (element=w610:string)
              n402 = Index Array(array=w603, index (row)=1, index (col)=14 ("disabled index (col)")) -> (element=w609:string)
              n403 = Index Array(array=w603, index (row)=1, index (col)=15 ("disabled index (col)")) -> (element=w604:string)
              n404 = global write "Global Variables.vi" "Setup"(w618) -> ()
              n405 = global write "Global Variables.vi" "PowerUp"(w613) -> ()
              n406 = global write "Global Variables.vi" "TachInputTest"(w610) -> ()
              n407 = global write "Global Variables.vi" "InclineTest"(w609) -> ()
              n408 = global write "Global Variables.vi" "ResistanceTest"(w604) -> ()
            }
            frame 10 {
              # "485"
              n409 = Index Array(array=w619, index (row)=11, index (col)=1 ("disabled index (col)")) -> (element=w634:string)
              n410 = Index Array(array=w619, index (row)=3, index (col)=5 ("disabled index (col)")) -> (element=w629:string)
              n411 = Index Array(array=w619, index (row)=1, index (col)=13 ("disabled index (col)")) -> (element=w626:string)
              n412 = Index Array(array=w619, index (row)=1, index (col)=14 ("disabled index (col)")) -> (element=w625:string)
              n413 = Index Array(array=w619, index (row)=1, index (col)=15 ("disabled index (col)")) -> (element=w620:string)
              n414 = global write "Global Variables.vi" "Setup"(w634) -> ()
              n415 = global write "Global Variables.vi" "PowerUp"(w629) -> ()
              n416 = global write "Global Variables.vi" "TachInputTest"(w626) -> ()
              n417 = global write "Global Variables.vi" "InclineTest"(w625) -> ()
              n418 = global write "Global Variables.vi" "ResistanceTest"(w620) -> ()
            }
            frame 12 {
              # "acc 485"
              n419 = Index Array(array=w635, index (row)=11, index (col)=1 ("disabled index (col)")) -> (element=w650:string)
              n420 = Index Array(array=w635, index (row)=3, index (col)=5 ("disabled index (col)")) -> (element=w645:string)
              n421 = Index Array(array=w635, index (row)=2, index (col)=13 ("disabled index (col)")) -> (element=w642:string)
              n422 = Index Array(array=w635, index (row)=1, index (col)=14 ("disabled index (col)")) -> (element=w641:string)
              n423 = Index Array(array=w635, index (row)=1, index (col)=15 ("disabled index (col)")) -> (element=w636:string)
              n424 = global write "Global Variables.vi" "Setup"(w650) -> ()
              n425 = global write "Global Variables.vi" "PowerUp"(w645) -> ()
              n426 = global write "Global Variables.vi" "TachInputTest"(w642) -> ()
              n427 = global write "Global Variables.vi" "InclineTest"(w641) -> ()
              n428 = global write "Global Variables.vi" "ResistanceTest"(w636) -> ()
            }
            frame 16 {
              # "acc powerboard???"
              n429 = Index Array(array=w651, index (row)=1, index (col)=2 ("disabled index (col)")) -> (element=w666:string)
              n430 = Index Array(array=w651, index (row)=1, index (col)=7 ("disabled index (col)")) -> (element=w661:string)
              n431 = Index Array(array=w651, index (row)=1, index (col)=7 ("disabled index (col)")) -> (element=w658:string)
              n432 = Index Array(array=w651, index (row)=1, index (col)=7 ("disabled index (col)")) -> (element=w657:string)
              n433 = Index Array(array=w651, index (row)=1, index (col)=7 ("disabled index (col)")) -> (element=w652:string)
              n434 = global write "Global Variables.vi" "Setup"(w666) -> ()
              n435 = global write "Global Variables.vi" "PowerUp"(w661) -> ()
              n436 = global write "Global Variables.vi" "TachInputTest"(w658) -> ()
              n437 = global write "Global Variables.vi" "InclineTest"(w657) -> ()
              n438 = global write "Global Variables.vi" "ResistanceTest"(w652) -> ()
            }
          }
        }
      }
    }
    frame "FITNESS_WT_MACH_DEVICE" {
      n439 = call "SpeedProtocol.vi"() -> ("output 1"=w670:i32)  [unwired: 9 in, 2 out]
      n440 = call "GradeProtocol.vi"() -> ("output 1"=w669:i32)  [unwired: 9 in, 2 out]
      n441 = Add(x=w670, y=w669) -> (x+y=w668:i32)
      n442 = case shown="4" w668 {
        tunnel: w667 -> [_ _ w671 w681]
        frame 0, Default {
        }
        frame 1 {
        }
        frame 2 {
          n443 = Index Array(array=w671, index (row)=3, index (col)=7 ("disabled index (col)")) -> (element=w675:string)
          n444 = Index Array(array=w671, index (row)=3, index (col)=2 ("disabled index (col)")) -> (element=w680:string)
          n445 = Index Array(array=w671, index (row)=1, index (col)=14 ("disabled index (col)")) -> (element=w672:string)
          n446 = global write "Global Variables.vi" "PowerUp"(w675) -> ()
          n447 = global write "Global Variables.vi" "Setup"(w680) -> ()
          n448 = global write "Global Variables.vi" "PWMTest"(w672) -> ()
        }
        frame 4 {
          n449 = Index Array(array=w681, index (row)=1, index (col)=2 ("disabled index (col)")) -> (element=w693:string)
          n450 = Index Array(array=w681, index (row)=1, index (col)=7 ("disabled index (col)")) -> (element=w688:string)
          n451 = Index Array(array=w681, index (row)=1, index (col)=7 ("disabled index (col)")) -> (element=w685:string)
          n452 = Index Array(array=w681, index (row)=1, index (col)=7 ("disabled index (col)")) -> (element=w684:string)
          n453 = global write "Global Variables.vi" "Setup"(w693) -> ()
          n454 = global write "Global Variables.vi" "PowerUp"(w688) -> ()
          n455 = global write "Global Variables.vi" "PWMTest"(w685) -> ()
          n456 = global write "Global Variables.vi" "InclineTest"(w684) -> ()
        }
      }
    }
    frame "FREE_STRIDER_DEVICE" {
      n457 = global read "Global Variables.vi" "MCU"() -> (w695:string)
      n458 = case shown="\"NRF51\"" w695 {
        tunnel: w694 -> [w697 w804]
        frame "PSOC", Default {
          n459 = call "GradeProtocol.vi"() -> ("output 1"=w698:i32)  [unwired: 9 in, 2 out]
          n460 = call "ResistanceProtocol.vi"() -> ("output 1"=w699:i32)  [unwired: 9 in, 2 out]
          n461 = call "DistanceProtocol.vi"() -> ("output 1"=w700:i32)  [unwired: 9 in, 2 out]
          n462 = Compound Arithmetic op=ADD(w698, w699, w700) -> (w696:i32)
          n463 = case shown="8" w696 {
            tunnel: w697 -> [_ _ w701 w711 w724 w740 w756 w772 w788]
            frame 0, Default {
            }
            frame 1 {
            }
            frame 3 {
              # "unknown"
              n464 = Index Array(array=w701, index (row)=3, index (col)=7 ("disabled index (col)")) -> (element=w705:string)
              n465 = Index Array(array=w701, index (row)=3, index (col)=2 ("disabled index (col)")) -> (element=w710:string)
              n466 = Index Array(array=w701, index (row)=1, index (col)=14 ("disabled index (col)")) -> (element=w702:string)
              n467 = global write "Global Variables.vi" "PowerUp"(w705) -> ()
              n468 = global write "Global Variables.vi" "Setup"(w710) -> ()
              n469 = global write "Global Variables.vi" "TachInputTest"(w702) -> ()
            }
            frame 5 {
              # "basic bike"
              n470 = Index Array(array=w711, index (row)=10, index (col)=5 ("disabled index (col)")) -> (element=w718:string)
              n471 = Index Array(array=w711, index (row)=8, index (col)=1 ("disabled index (col)")) -> (element=w723:string)
              n472 = Index Array(array=w711, index (row)=1, index (col)=13 ("disabled index (col)")) -> (element=w715:string)
              n473 = Index Array(array=w711, index (row)=1, index (col)=15 ("disabled index (col)")) -> (element=w714:string)
              n474 = global write "Global Variables.vi" "PowerUp"(w718) -> ()
              n475 = global write "Global Variables.vi" "Setup"(w723) -> ()
              n476 = global write "Global Variables.vi" "ResistanceTest"(w714) -> ()
              n477 = global write "Global Variables.vi" "TachInputTest"(w715) -> ()
            }
            frame 6 {
              # "analog"
              n478 = Index Array(array=w724, index (row)=10, index (col)=1 ("disabled index (col)")) -> (element=w739:string)
              n479 = Index Array(array=w724, index (row)=2, index (col)=5 ("disabled index (col)")) -> (element=w734:string)
              n480 = Index Array(array=w724, index (row)=1, index (col)=13 ("disabled index (col)")) -> (element=w731:string)
              n481 = Index Array(array=w724, index (row)=1, index (col)=14 ("disabled index (col)")) -> (element=w730:string)
              n482 = Index Array(array=w724, index (row)=1, index (col)=15 ("disabled index (col)")) -> (element=w725:string)
              n483 = global write "Global Variables.vi" "Setup"(w739) -> ()
              n484 = global write "Global Variables.vi" "PowerUp"(w734) -> ()
              n485 = global write "Global Variables.vi" "TachInputTest"(w731) -> ()
              n486 = global write "Global Variables.vi" "InclineTest"(w730) -> ()
              n487 = global write "Global Variables.vi" "ResistanceTest"(w725) -> ()
            }
            frame 8 {
              # "accelerometer"
              n488 = Index Array(array=w740, index (row)=19, index (col)=1 ("disabled index (col)")) -> (element=w755:string)
              n489 = Index Array(array=w740, index (row)=19, index (col)=5 ("disabled index (col)")) -> (element=w750:string)
              n490 = Index Array(array=w740, index (row)=2, index (col)=13 ("disabled index (col)")) -> (element=w747:string)
              n491 = Index Array(array=w740, index (row)=1, index (col)=14 ("disabled index (col)")) -> (element=w746:string)
              n492 = Index Array(array=w740, index (row)=1, index (col)=15 ("disabled index (col)")) -> (element=w741:string)
              n493 = global write "Global Variables.vi" "Setup"(w755) -> ()
              n494 = global write "Global Variables.vi" "PowerUp"(w750) -> ()
              n495 = global write "Global Variables.vi" "TachInputTest"(w747) -> ()
              n496 = global write "Global Variables.vi" "InclineTest"(w746) -> ()
              n497 = global write "Global Variables.vi" "ResistanceTest"(w741) -> ()
            }
            frame 10 {
              # "485"
              n498 = Index Array(array=w756, index (row)=11, index (col)=1 ("disabled index (col)")) -> (element=w771:string)
              n499 = Index Array(array=w756, index (row)=3, index (col)=5 ("disabled index (col)")) -> (element=w766:string)
              n500 = Index Array(array=w756, index (row)=1, index (col)=13 ("disabled index (col)")) -> (element=w763:string)
              n501 = Index Array(array=w756, index (row)=1, index (col)=14 ("disabled index (col)")) -> (element=w762:string)
              n502 = Index Array(array=w756, index (row)=1, index (col)=15 ("disabled index (col)")) -> (element=w757:string)
              n503 = global write "Global Variables.vi" "Setup"(w771) -> ()
              n504 = global write "Global Variables.vi" "PowerUp"(w766) -> ()
              n505 = global write "Global Variables.vi" "TachInputTest"(w763) -> ()
              n506 = global write "Global Variables.vi" "InclineTest"(w762) -> ()
              n507 = global write "Global Variables.vi" "ResistanceTest"(w757) -> ()
            }
            frame 12 {
              # "acc 485"
              n508 = Index Array(array=w772, index (row)=11, index (col)=1 ("disabled index (col)")) -> (element=w787:string)
              n509 = Index Array(array=w772, index (row)=3, index (col)=5 ("disabled index (col)")) -> (element=w782:string)
              n510 = Index Array(array=w772, index (row)=2, index (col)=13 ("disabled index (col)")) -> (element=w779:string)
              n511 = Index Array(array=w772, index (row)=1, index (col)=14 ("disabled index (col)")) -> (element=w778:string)
              n512 = Index Array(array=w772, index (row)=1, index (col)=15 ("disabled index (col)")) -> (element=w773:string)
              n513 = global write "Global Variables.vi" "Setup"(w787) -> ()
              n514 = global write "Global Variables.vi" "PowerUp"(w782) -> ()
              n515 = global write "Global Variables.vi" "TachInputTest"(w779) -> ()
              n516 = global write "Global Variables.vi" "InclineTest"(w778) -> ()
              n517 = global write "Global Variables.vi" "ResistanceTest"(w773) -> ()
            }
            frame 16 {
              # "acc powerboard???"
              n518 = Index Array(array=w788, index (row)=1, index (col)=2 ("disabled index (col)")) -> (element=w803:string)
              n519 = Index Array(array=w788, index (row)=1, index (col)=7 ("disabled index (col)")) -> (element=w798:string)
              n520 = Index Array(array=w788, index (row)=1, index (col)=7 ("disabled index (col)")) -> (element=w795:string)
              n521 = Index Array(array=w788, index (row)=1, index (col)=7 ("disabled index (col)")) -> (element=w794:string)
              n522 = Index Array(array=w788, index (row)=1, index (col)=7 ("disabled index (col)")) -> (element=w789:string)
              n523 = global write "Global Variables.vi" "Setup"(w803) -> ()
              n524 = global write "Global Variables.vi" "PowerUp"(w798) -> ()
              n525 = global write "Global Variables.vi" "TachInputTest"(w795) -> ()
              n526 = global write "Global Variables.vi" "InclineTest"(w794) -> ()
              n527 = global write "Global Variables.vi" "ResistanceTest"(w789) -> ()
            }
          }
        }
        frame "NRF51" {
          n528 = call "GradeProtocol.vi"() -> ("output 1"=w806:i32)  [unwired: 9 in, 2 out]
          n529 = call "ResistanceProtocol.vi"() -> ("output 1"=w807:i32)  [unwired: 9 in, 2 out]
          n530 = call "DistanceProtocol.vi"() -> ("output 1"=w808:i32)  [unwired: 9 in, 2 out]
          n531 = call "maintenanceBLE.vi"("Shared_strings"=w804) -> ()  [unwired: 11 in]
          n532 = Compound Arithmetic op=ADD(w806, w807, w808) -> (w805:i32)
          n533 = case shown="10" w805 {
            tunnel: w804 -> [_ _ w809 w819 w832 w848 w864 w880 w896]
            frame 0, Default {
            }
            frame 1 {
            }
            frame 3 {
              # "unknown"
              n534 = Index Array(array=w809, index (row)=3, index (col)=7 ("disabled index (col)")) -> (element=w813:string)
              n535 = Index Array(array=w809, index (row)=3, index (col)=2 ("disabled index (col)")) -> (element=w818:string)
              n536 = Index Array(array=w809, index (row)=1, index (col)=14 ("disabled index (col)")) -> (element=w810:string)
              n537 = global write "Global Variables.vi" "PowerUp"(w813) -> ()
              n538 = global write "Global Variables.vi" "Setup"(w818) -> ()
              n539 = global write "Global Variables.vi" "TachInputTest"(w810) -> ()
            }
            frame 5 {
              # "basic bike"
              n540 = Index Array(array=w819, index (row)=10, index (col)=5 ("disabled index (col)")) -> (element=w826:string)
              n541 = Index Array(array=w819, index (row)=8, index (col)=1 ("disabled index (col)")) -> (element=w831:string)
              n542 = Index Array(array=w819, index (row)=1, index (col)=13 ("disabled index (col)")) -> (element=w823:string)
              n543 = Index Array(array=w819, index (row)=1, index (col)=15 ("disabled index (col)")) -> (element=w822:string)
              n544 = global write "Global Variables.vi" "PowerUp"(w826) -> ()
              n545 = global write "Global Variables.vi" "Setup"(w831) -> ()
              n546 = global write "Global Variables.vi" "ResistanceTest"(w822) -> ()
              n547 = global write "Global Variables.vi" "TachInputTest"(w823) -> ()
            }
            frame 6 {
              # "analog"
              n548 = Index Array(array=w832, index (row)=10, index (col)=1 ("disabled index (col)")) -> (element=w847:string)
              n549 = Index Array(array=w832, index (row)=2, index (col)=5 ("disabled index (col)")) -> (element=w842:string)
              n550 = Index Array(array=w832, index (row)=1, index (col)=13 ("disabled index (col)")) -> (element=w839:string)
              n551 = Index Array(array=w832, index (row)=1, index (col)=14 ("disabled index (col)")) -> (element=w838:string)
              n552 = Index Array(array=w832, index (row)=1, index (col)=15 ("disabled index (col)")) -> (element=w833:string)
              n553 = global write "Global Variables.vi" "Setup"(w847) -> ()
              n554 = global write "Global Variables.vi" "PowerUp"(w842) -> ()
              n555 = global write "Global Variables.vi" "TachInputTest"(w839) -> ()
              n556 = global write "Global Variables.vi" "InclineTest"(w838) -> ()
              n557 = global write "Global Variables.vi" "ResistanceTest"(w833) -> ()
            }
            frame 8 {
              # "accelerometer"
              n558 = Index Array(array=w848, index (row)=19, index (col)=1 ("disabled index (col)")) -> (element=w863:string)
              n559 = Index Array(array=w848, index (row)=19, index (col)=5 ("disabled index (col)")) -> (element=w858:string)
              n560 = Index Array(array=w848, index (row)=2, index (col)=13 ("disabled index (col)")) -> (element=w855:string)
              n561 = Index Array(array=w848, index (row)=1, index (col)=14 ("disabled index (col)")) -> (element=w854:string)
              n562 = Index Array(array=w848, index (row)=1, index (col)=15 ("disabled index (col)")) -> (element=w849:string)
              n563 = global write "Global Variables.vi" "Setup"(w863) -> ()
              n564 = global write "Global Variables.vi" "PowerUp"(w858) -> ()
              n565 = global write "Global Variables.vi" "TachInputTest"(w855) -> ()
              n566 = global write "Global Variables.vi" "InclineTest"(w854) -> ()
              n567 = global write "Global Variables.vi" "ResistanceTest"(w849) -> ()
            }
            frame 10 {
              # "485"
              n568 = Index Array(array=w864, index (row)=11, index (col)=1 ("disabled index (col)")) -> (element=w879:string)
              n569 = Index Array(array=w864, index (row)=3, index (col)=5 ("disabled index (col)")) -> (element=w874:string)
              n570 = Index Array(array=w864, index (row)=1, index (col)=13 ("disabled index (col)")) -> (element=w871:string)
              n571 = Index Array(array=w864, index (row)=1, index (col)=14 ("disabled index (col)")) -> (element=w870:string)
              n572 = Index Array(array=w864, index (row)=1, index (col)=15 ("disabled index (col)")) -> (element=w865:string)
              n573 = global write "Global Variables.vi" "Setup"(w879) -> ()
              n574 = global write "Global Variables.vi" "PowerUp"(w874) -> ()
              n575 = global write "Global Variables.vi" "TachInputTest"(w871) -> ()
              n576 = global write "Global Variables.vi" "InclineTest"(w870) -> ()
              n577 = global write "Global Variables.vi" "ResistanceTest"(w865) -> ()
            }
            frame 12 {
              # "acc 485"
              n578 = Index Array(array=w880, index (row)=11, index (col)=1 ("disabled index (col)")) -> (element=w895:string)
              n579 = Index Array(array=w880, index (row)=3, index (col)=5 ("disabled index (col)")) -> (element=w890:string)
              n580 = Index Array(array=w880, index (row)=2, index (col)=13 ("disabled index (col)")) -> (element=w887:string)
              n581 = Index Array(array=w880, index (row)=1, index (col)=14 ("disabled index (col)")) -> (element=w886:string)
              n582 = Index Array(array=w880, index (row)=1, index (col)=15 ("disabled index (col)")) -> (element=w881:string)
              n583 = global write "Global Variables.vi" "Setup"(w895) -> ()
              n584 = global write "Global Variables.vi" "PowerUp"(w890) -> ()
              n585 = global write "Global Variables.vi" "TachInputTest"(w887) -> ()
              n586 = global write "Global Variables.vi" "InclineTest"(w886) -> ()
              n587 = global write "Global Variables.vi" "ResistanceTest"(w881) -> ()
            }
            frame 16 {
              # "acc powerboard???"
              n588 = Index Array(array=w896, index (row)=1, index (col)=2 ("disabled index (col)")) -> (element=w911:string)
              n589 = Index Array(array=w896, index (row)=1, index (col)=7 ("disabled index (col)")) -> (element=w906:string)
              n590 = Index Array(array=w896, index (row)=1, index (col)=7 ("disabled index (col)")) -> (element=w903:string)
              n591 = Index Array(array=w896, index (row)=1, index (col)=7 ("disabled index (col)")) -> (element=w902:string)
              n592 = Index Array(array=w896, index (row)=1, index (col)=7 ("disabled index (col)")) -> (element=w897:string)
              n593 = global write "Global Variables.vi" "Setup"(w911) -> ()
              n594 = global write "Global Variables.vi" "PowerUp"(w906) -> ()
              n595 = global write "Global Variables.vi" "TachInputTest"(w903) -> ()
              n596 = global write "Global Variables.vi" "InclineTest"(w902) -> ()
              n597 = global write "Global Variables.vi" "ResistanceTest"(w897) -> ()
            }
          }
        }
      }
    }
    frame "ROWER_DEVICE" {
      n598 = call "SpeedProtocol.vi"() -> ("output 1"=w912:i32)  [unwired: 9 in, 2 out]
      n599 = case shown="1" w912 {
        tunnel: w913 -> [_ w914 w924 _]
        frame 0, Default {
        }
        frame 1 {
          n600 = call "maintenanceBLE.vi"("Shared_strings"=w914) -> ()  [unwired: 11 in]
          n601 = Index Array(array=w914, index (row)=15, index (col)=5 ("disabled index (col)")) -> (element=w918:string)
          n602 = Index Array(array=w914, index (row)=15, index (col)=1 ("disabled index (col)")) -> (element=w923:string)
          n603 = Index Array(array=w914, index (row)=1, index (col)=13 ("disabled index (col)")) -> (element=w915:string)
          n604 = global write "Global Variables.vi" "PowerUp"(w918) -> ()
          n605 = global write "Global Variables.vi" "Setup"(w923) -> ()
          n606 = global write "Global Variables.vi" "TachInputTest"(w915) -> ()
        }
        frame 2 {
          # "tablet console"
          n607 = Index Array(array=w924, index (row)=16, index (col)=7 ("disabled index (col)")) -> (element=w928:string)
          n608 = Index Array(array=w924, index (row)=20, index (col)=2 ("disabled index (col)")) -> (element=w933:string)
          n609 = global write "Global Variables.vi" "PowerUp"(w928) -> ()
          n610 = global write "Global Variables.vi" "Setup"(w933) -> ()
          n611 = Index Array(array=w924, index (row)=1, index (col)=15 ("disabled index (col)")) -> (element=w925:string)
          n612 = global write "Global Variables.vi" "TachInputTest"(w925) -> ()
        }
        frame 4 {
        }
      }
    }
  }
